vi "Convert FXP 24.1 to Integer 24.1.vi"() -> (1 "normv[M..1]":i32[](array[numeric]), 2 "^normk[M..1]":i32[](array[numeric]), 3 "normk[M..1]":i32[](array[numeric]))   [LabVIEW 2023]
doc: "Demonstrates how to use the Fixed-Point Tools VIs to obtain the integer coefficients of a notch filter with a normalized sections type of the lattice autoregressive-moving average (ARMA) structure."
uses:
  <vilib>/addons/Digital Filter Design/_Objects.llb/DFD Quantization Settings.ctl
  <vilib>/addons/Digital Filter Design/_Objects.llb/DFD Quantization Sources.ctl
  <vilib>/addons/Digital Filter Design/Design.llb/DFD IIR Notch Peak Design by Q.vi
  <vilib>/addons/Digital Filter Design/FXPLib.llb/DFD FXP to I32 (vector).vi
  <vilib>/addons/Digital Filter Design/NI_DigFilterLicensed.lvlib
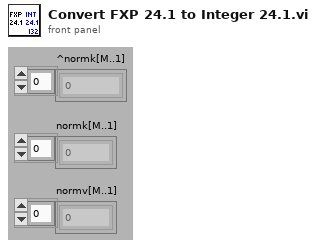
[diagram p1: front panel]
types:
  T1 = typedef "NI_DigFilterLicensed.lvlib/DFD Quantization Settings.ctl" = cluster{"source":T2, "wl":i16, "iwl":i16, "overflow mode":enum16{"Saturation", "Wrap"}, "rounding mode":enum16{"Nearest", "Truncation"}, "signed?":bool}
  T2 = typedef "NI_DigFilterLicensed.lvlib/DFD Quantization Sources.ctl" = u16
  T3 = typedef "NI_DigFilterLicensed.lvlib/DFD Filter Obj.ctl" = cluster{"mSRate_Fs":dbl, "mSRate_Version":string, "mSRate_Comments":string, "mSRate_OrgCoef":T4, "mSRate_CurCoef":T4, "mSRate_Quantized?":bool, "mSRate_QCoef":T4, "mSRate_QSettings":T6[], "mSRate_Order":i32, "mSRate_Scaling":cluster{"mSRate_ScaleByPowerOf2?":bool, "mSRate_ScaleType":T8}}
  T4 = typedef "NI_DigFilterLicensed.lvlib/DFD Filter Coef.ctl" = cluster{"type":T5, "gain":dbl, "coef a (k)":dbl[], "coef b (v)":dbl[]}
  T5 = typedef "NI_DigFilterLicensed.lvlib/DFD Filter Structure Type Selector.ctl" = enum16{"Undefined", "FIR Direct Form", "FIR Direct Form Transposed", "FIR Symmetric", "FIR Antisymmetric", "IIR Direct Form I", "IIR Direct Form I Transposed", "IIR Direct Form II", "IIR Direct Form II Transposed", "IIR Cascaded Second Order Sections Form I", "IIR Cascaded Second Order Sections Form I Transposed", "IIR Cascaded Second Order Sections Form II", "IIR Cascaded Second Order Sections Form II Transposed", "Lattice Allpass (basic sections)", "Lattice Allpass (one multiplier sections)", "Lattice Allpass (normalized sections)", "Lattice AR (basic sections)", "Lattice AR (one multiplier sections)", "Lattice AR (normalized sections)", "Lattice MA (minimum phase)", "Lattice MA (maximum phase)", "Lattice ARMA (basic sections)", "Lattice ARMA (one multiplier sections)", "Lattice ARMA (normalized sections)"}
  T6 = typedef "NI_DigFilterLicensed.lvlib/dfd_Internal Quantization Settings.ctl" = cluster{"source":T7, "wl":i16, "iwl":i16, "overflow mode":enum16{"Saturation", "Wrap"}, "rounding mode":enum16{"Nearest", "Truncation"}, "signed?":bool}
  T7 = typedef "NI_DigFilterLicensed.lvlib/dfd_Internal Quantization Srcs.ctl" = u16
  T8 = typedef "NI_DigFilterLicensed.lvlib/DFD Coef Norm Type.ctl" = enum16{"No Norm", "Time Domain 1-Norm", "Time Domain 2-Norm", "Time Domain Inf-Norm"}
  T9 = cluster{"structure type":u16, "reflection coefficients":dbl[], "ladder coefficients":dbl[], "gain":dbl}
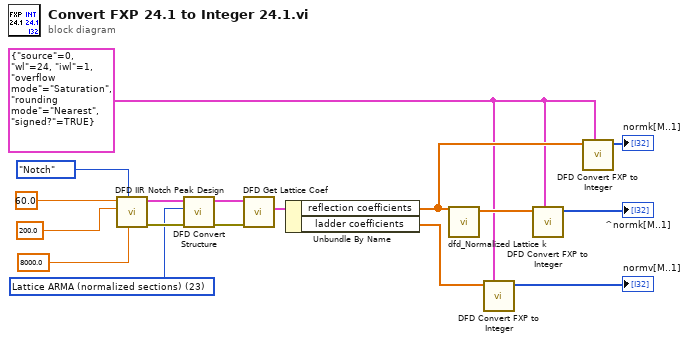
[diagram p0: block diagram]
diagram:
  w1 = u16 23 items=["FIR Direct Form"=1, "FIR Direct Form Transposed"=2, "FIR Symmetric"=3, "FIR Antisymmetric"=4, "IIR Direct Form I"=5, "IIR Direct Form I Transposed"=6, "IIR Direct Form II"=7, "IIR Direct Form II Transposed"=8, "IIR Cascaded Second-Order Sections Form I"=9, "IIR Cascaded Second-Order Sections Form I Transposed"=10, "IIR Cascaded Second-Order Sections Form II"=11, "IIR Cascaded Second-Order Sections Form II Transposed"=12, "Lattice Allpass (basic sections)"=13, "Lattice Allpass (one multiplier sections)"=14, "Lattice Allpass (normalized sections)"=15, "Lattice AR (basic sections)"=16, "Lattice AR (one multiplier sections)"=17, "Lattice AR (normalized sections)"=18, "Lattice MA (minimum phase)"=19, "Lattice MA (maximum phase)"=20, "Lattice ARMA (basic sections)"=21, "Lattice ARMA (one multiplier sections)"=22, "Lattice ARMA (normalized sections)"=23] ("target structure")
  w4 = T1 {"source"=0, "wl"=24, "iwl"=1, "overflow mode"=enum."Saturation", "rounding mode"=enum."Nearest", "signed?"=TRUE} ("Coefficient quantizer")
  n1 = call-poly <vilib>:"DFD IIR Notch Peak Design.vi"("fs [Hz]"=8000.0, "filter type"=enum16{"Notch", "Peak"}."Notch", "Q factor"=200.0, "f0 [Hz]"=60.0) -> ("error out"=w12:errorcluster, "filter out"=w13:T3)  [unwired: 1 in, 5 out]
  n2 = call <vilib>:"DFD Convert Structure.vi"("error in (no error)"=w12, "target structure"=w1, "filter in"=w13) -> ("error out"=w2:errorcluster, "filter out"=w3:T3)  [unwired: 7 out]
  n3 = call <vilib>:"DFD Get Lattice Coef.vi"("error in (no error)"=w2, "filter in"=w3) -> ("lattice coef"=w10:T9)  [unwired: 9 out]
  n4 = Unbundle By Name(w10) -> ("reflection coefficients"=w8:dbl[], "ladder coefficients"=w5:dbl[])
  n5 = call <vilib>:"dfd_Normalized Lattice k.vi"("k"=w8) -> ("^k"=w9:dbl[])  [unwired: 10 out]
  n6 = call-poly <vilib>:"DFD Convert FXP to Integer.vi"("quantization settings"=w4, "FXP values"=w5) -> ("I32 values"=→"normv[M..1]":i32[])  [unwired: 1 in, 8 out]
  n7 = call-poly <vilib>:"DFD Convert FXP to Integer.vi"("quantization settings"=w4, "FXP values"=w9) -> ("I32 values"=→"^normk[M..1]":i32[])  [unwired: 1 in, 8 out]
  n8 = call-poly <vilib>:"DFD Convert FXP to Integer.vi"("quantization settings"=w4, "FXP values"=w8) -> ("I32 values"=→"normk[M..1]":i32[])  [unwired: 1 in, 8 out]
